vi "Degrees to Radians (Scalar SGL).vi"(3 "angle (deg)":sgl) -> (1 "angle (rad)":sgl)   [LabVIEW 2020, in "NI_AngleManipulation.lvlib"]
doc: "Converts an angle from degrees to radians."
uses:
  <vilib>/Utility/AngleManip/NI_AngleManipulation.lvlib
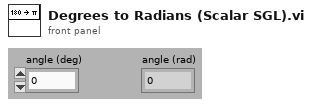
[diagram p1: front panel]
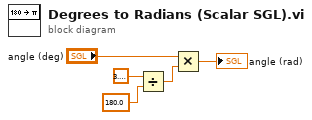
[diagram p0: block diagram]
diagram:
  n1 = Divide(x=sgl 3.1415927, y=sgl 180.0) -> (x/y=w2:sgl)
  n2 = Multiply(x="angle (deg)", y=w2) -> (x*y=→"angle (rad)":sgl)
